vi "Configuracao.Variaveis.vi"() -> ()   [LabVIEW 2019]
panel:
  in  "Medicoes":string[][](array[string])
  in  "Medicao":dbl
  out "Medir":bool
  in  "Cluster":T1
  in  "TipoMedicao":string
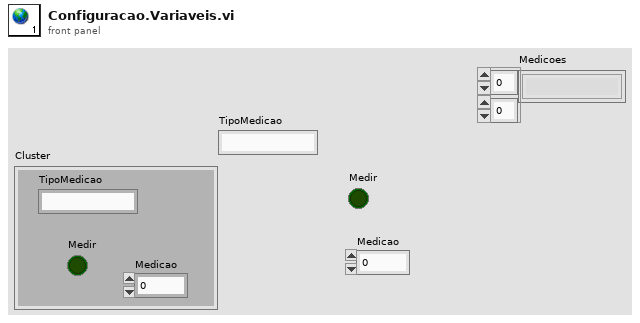
[diagram p1: front panel]
types:
  T1 = cluster{"TipoMedicao":string, "Medir":bool, "Medicao":dbl}
diagram:
